vi "Group Data Type.vi"(8 "error in (no error)":errorcluster, 11 "StringGroup in":refnum<class "StringGroup.lvclass">) -> (0 "error out":errorcluster, 2 "Group Data Type":T1, 3 "StringGroup out":refnum<class "StringGroup.lvclass">)   [LabVIEW 2020, in "Vecto.lvlib" / "StringGroup.lvclass"]
uses:
  StringGroup.lvclass
  Group Data Type.ctl
  StringGroup.lvclass/StringGroup.ctl
  Vecto.lvlib
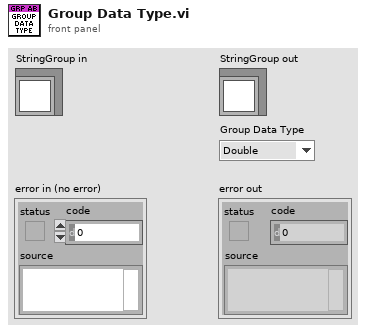
[diagram p1: front panel]
types:
  T1 = typedef "Vecto.lvlib/Group Data Type.ctl" = enum16{"Double", "String"}
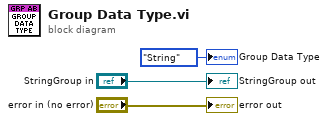
[diagram p0: block diagram]
diagram:
  "error out" <- "error in (no error)"
  "StringGroup out" <- "StringGroup in"
  "Group Data Type" <- Group_Data_Type."String" ("Group Data Type")
